vi "Remove Invalid DMAs.vi"(8 "error in (no error)":errorcluster, 9 "invalid DMA channels":T1[](array[typedef]) {"Data Type" format="%.0x"}, 10 "section name":string, 11 "item ref in":T3 format="%.0x") -> (0 "error out":errorcluster, 3 "item ref out":T3 format="%.0x")   [LabVIEW 2018, in "FPGA Addon System Explorer.lvlib"]
uses:
  FPGA Addon System Explorer.lvlib
  <vilib>/NI Veristand/Custom Device API/Custom Device Item Ref.ctl
  Addon Shared/Types/DMA Information.ctl
  Addon Shared/Types/Data Type.ctl
  <vilib>/NI Veristand/Custom Device Tools/Custom Device Utility Library/NI VeriStand - Search for Item by Name.vi
  <vilib>/NI Veristand/Custom Device Tools/Custom Device Utility Library/Custom Device Utility Library.lvlib
  <vilib>/NI Veristand/Custom Device API/Custom Device API.lvlib
  Addon Shared/FPGA Addon Shared.lvlib
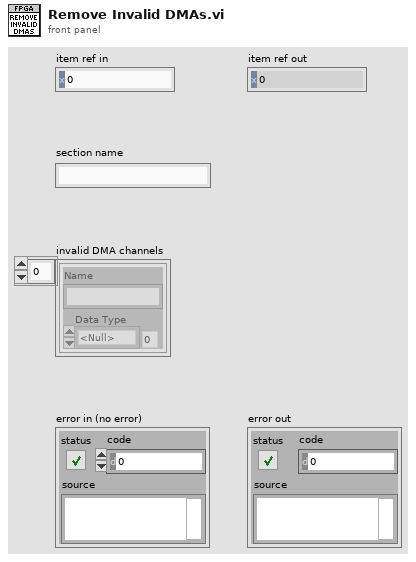
[diagram p1: front panel]
types:
  T1 = typedef "FPGA Addon Shared.lvlib/DMA Information.ctl" = cluster{"Name":string, "Data Type":T2}
  T2 = typedef "FPGA Addon Shared.lvlib/Data Type.ctl" = enum8{"<Null>", "I8", "I16", "I32", "I64", "U8", "U16", "U32", "U64", "SGL", "Boolean", "Analog PWM In Settings", "Analog PWM In", "Digital PWM In Settings", "Digital PWM In", "Digital PWM Out", "Sine Out", "FXP+/-24.5", "FXP+/-16.5", "FXP+/-32.8", "FXP+/-64.32", "FXP+/-16.7", "FXP+/-20.5", "FXP+/-27.5", "FXP+/-32.16", "FXP+16.3", "FXP+18.3", "Digital Static In", "Digital Static Out", "Digital Static In Settings", "Digital WSS Out", "Quad Encoder Settings", "Quad Encoder In", "Group"}
  T3 = typedef "Custom Device API.lvlib/Custom Device Item Ref.ctl" = u64
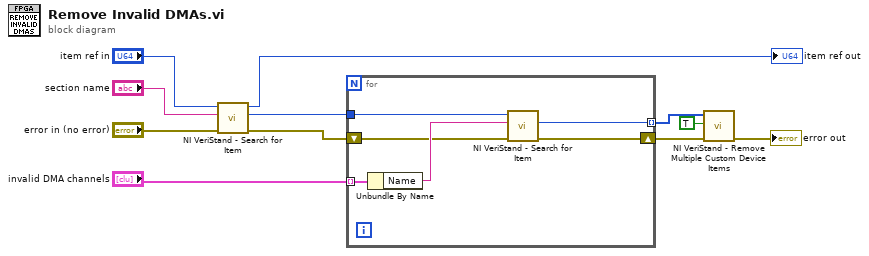
[diagram p0: block diagram]
diagram:
  n1 = call-poly <vilib>:"NI VeriStand - Search for Item.vi"("error in"="error in (no error)", "Item Name"="section name", "Section Ref in"="item ref in") -> ("error out"=w8:errorcluster, "Item Ref"=w7:T3, "Section Ref out"=→"item ref out":T3)  [unwired: 5 in, 1 out]
  n2 = for {
    tunnel: w7 -> [w17]
    tunnel: "invalid DMA channels" -> [w16] mode=indexing
    shift-right: [w13] -> w10
    shift-left: w8 -> [w14]
    tunnel: [w12] -> w9 mode=indexing
    n3 = Unbundle By Name(w16) -> ("Name"=w15:string)
    n4 = call-poly <vilib>:"NI VeriStand - Search for Item.vi"("error in"=w14, "Item Name"=w15, "Section Ref in"=w17) -> ("error out"=w13:errorcluster, "Item Ref"=w12:T3)  [unwired: 5 in, 2 out]
  }
  n5 = call <vilib>:"NI VeriStand - Remove Multiple Custom Device Items.vi"("error in (no error)"=w10, "Force Delete (F)"=TRUE, "Item Refs in"=w9) -> ("error out"=→"error out":errorcluster)  [unwired: 7 in, 1 out]
